vi "InterfaceByViServer_Example1.vi"() -> ()   [LabVIEW 2012]
uses:
  Base_class/Base.lvclass
  Sub_class/Sub.lvclass
  Leaf_class/Leaf.lvclass
  Interface1_Interface/Interface1.lvclass
panel:
  out "String 4":string
  out "error out 4":errorcluster
  out "error out 3":errorcluster
  out "String 3":string
  out "String 2":string
  out "error out 2":errorcluster
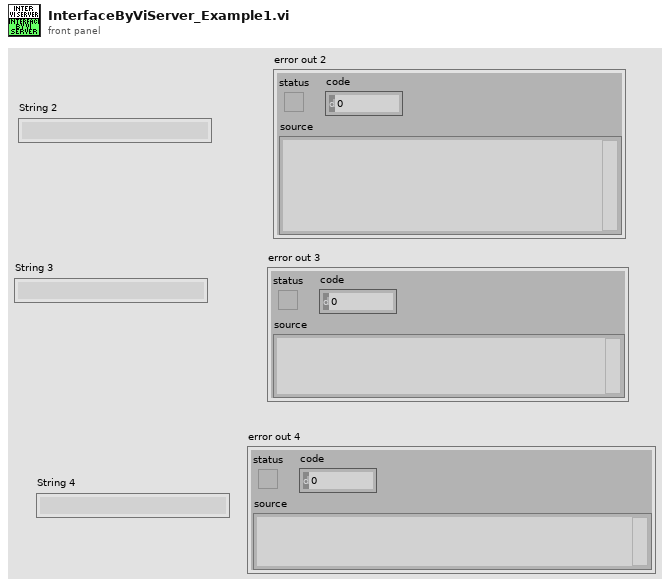
[diagram p1: front panel]
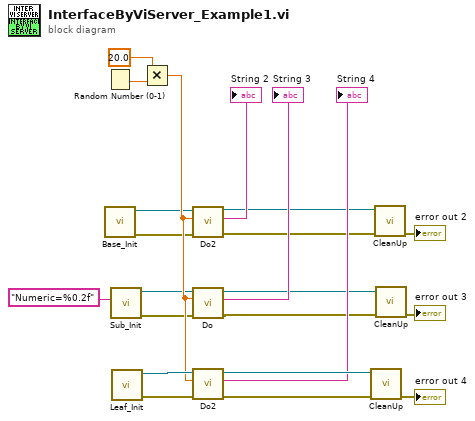
[diagram p0: block diagram]
diagram:
  n1 = Random Number (0-1)() -> (number: 0 to 1=w22:dbl)
  n2 = call "Base_Init.vi"() -> ("error out"=w9:errorcluster, "object out"=w10:refnum<class "Base.lvclass">)  [unwired: 10 in]
  n3 = call "Sub_Init.vi"("String"="Numeric=%0.2f") -> ("error out"=w6:errorcluster, "object out"=w5:refnum<class "Sub.lvclass">)  [unwired: 9 in]
  n4 = call "Leaf_Init.vi"() -> ("error out"=w18:errorcluster, "object out"=w17:refnum<class "Leaf.lvclass">)  [unwired: 10 in]
  n5 = Multiply(x=20.0, y=w22) -> (x*y=w16:dbl)
  n6 = call "Do2.vi"("error in (no error)"=w9, "Numeric"=w16, "Interface In"=w10) -> ("error out"=w8:errorcluster, "String"=→"String 2":string, "Interface Out"=w7:refnum<class "Base.lvclass">)  [unwired: 6 in]
  n7 = call "Do.vi"("error in (no error)"=w6, "Numeric"=w16, "Interface In"=w5) -> ("error out"=w3:errorcluster, "String"=→"String 3":string, "Interface Out"=w4:refnum<class "Sub.lvclass">)  [unwired: 6 in]
  n8 = call "Do2.vi"("error in (no error)"=w18, "Numeric"=w16, "Interface In"=w17) -> ("error out"=w15:errorcluster, "String"=→"String 4":string, "Interface Out"=w14:refnum<class "Leaf.lvclass">)  [unwired: 6 in]
  n9 = call-dynamic "CleanUp.vi"("error in (no error)"=w15, "Object in"=w14) -> ("error out"=→"error out 4":errorcluster)  [unwired: 8 in, 1 out]
  n10 = call-dynamic "CleanUp.vi"("error in (no error)"=w8, "object in"=w7) -> ("error out"=→"error out 2":errorcluster)  [unwired: 8 in, 1 out]
  n11 = call-dynamic "CleanUp.vi"("error in (no error)"=w3, "Object in"=w4) -> ("error out"=→"error out 3":errorcluster)  [unwired: 8 in, 1 out]
